vi "Store Value in TDMS.vi"(6 "Value":variant, 7 "Prefix":string, 8 "Error In":errorcluster, 9 "channel name":string, 10 "group name":string, 11 "tdms file":refnum<k34>) -> (0 "Error Out":errorcluster, 1 "channel name out":string, 2 "group name out":string, 3 "tdms file out":refnum<k34>)   [LabVIEW 2019]
uses:
  <vilib>/Utility/Data Type/Type Definitions/Data Type.ctl
  <vilib>/Utility/Data Type/NI_Data Type.lvlib
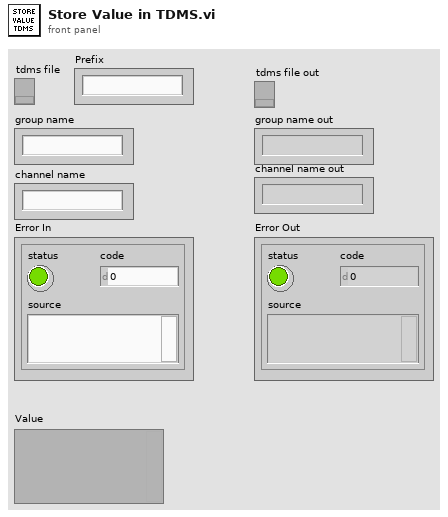
[diagram p1: front panel]
types:
  T1 = typedef "NI_Data Type.lvlib/Data Type.ctl" = enum8{"Invalid Type", "Void", "I8", "I16", "I32", "I64", "U8", "U16", "U32", "U64", "Single Float", "Double Float", "Extended Float", "Single Complex", "Double Complex", "Extended Complex", "Enum U8", "Enum U16", "Enum U32", "Enum U64", "Single Float With Unit", "Double Float With Unit", "Extended Float With Unit", "Single Complex with Unit", "Double Complex with Unit", "Extended Complex with Unit", "Boolean", "String", "Path", "Picture", "Tag", "Array", "Cluster", "Variant", "LV Variant", "Waveform", "Timestamp", "Digital Waveform", "Digital Data", "ExpressData", "Refnum", "External Data", "VI", "Poly VI", "LabVIEW Class Instance", "Fixed Point", "Set Collection", "Map Collection"}
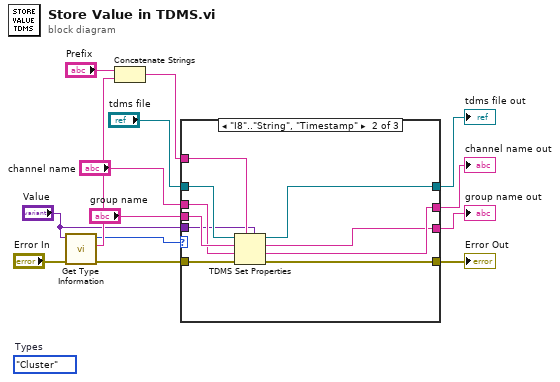
[diagram p0: block diagram]
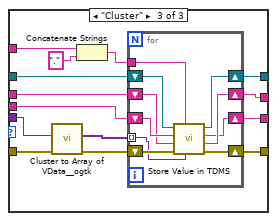
[diagram p3: hidden frame]
diagram:
  (unwired) Data_Type."Cluster"  # Types
  n1 = call <vilib>:"Get Type Information.vi"("error in (no error)"="Error In", "variant"="Value") -> ("error out"=w5:errorcluster, "name"=w7:string, "type"=w4:T1)  [unwired: 5 in, 2 out]
  n2 = Concatenate Strings("Prefix", w7) -> (w2:string)
  n3 = case shown="\"I8\"..\"String\", \"Timestamp\"" w4 {
    tunnel: "tdms file" -> [w18 w28 w42]
    tunnel: [w18 w27 w36] -> w13
    tunnel: "group name" -> [w16 w26 w41]
    tunnel: "channel name" -> [w15 w25 w40]
    tunnel: [w15 w24 w38] -> w10
    tunnel: [w16 w23 w39] -> w9
    tunnel: w5 -> [w17 w22 w30]
    tunnel: [w17 w21 w37] -> w8
    tunnel: w2 -> [_ w20 w35]
    tunnel: "Value" -> [_ w19 w32]
    frame "Invalid Type", Default {
    }
    frame "I8".."String", "Timestamp" {
      n4 = TDMS Set Properties(5:w19, 7:w20, 8:w22, 9:w25, 10:w26, 11:w28) -> (0:w21:errorcluster, 1:w24:string, 2:w23:string, 3:w27:refnum<k34>)
    }
    frame "Cluster" {
      n5 = call <userlib>:"Cluster to Array of VData__ogtk.vi"("error in (no error)"=w30, "Cluster"=w32) -> ("error out"=w29:errorcluster, "Array of VData"=w31:variant[])  [unwired: 8 in]
      n6 = Concatenate Strings(w35, "." ("string")) -> (w33:string)
      n7 = for {
        shift-right: [w49] -> w37
        shift-left: w29 -> [w51]
        shift-right: [w50] -> w36
        shift-left: w42 -> [w52]
        shift-right: [w45] -> w39
        shift-left: w41 -> [w48]
        shift-right: [w46] -> w38
        shift-left: w40 -> [w47]
        tunnel: w31 -> [w44] mode=indexing
        tunnel: w33 -> [w43]
        n8 = call "Store Value in TDMS.vi"("Value"=w44, "Prefix"=w43, "Error In"=w51, "channel name"=w47, "group name"=w48, "tdms file"=w52) -> ("Error Out"=w49:errorcluster, "channel name out"=w46:string, "group name out"=w45:string, "tdms file out"=w50:refnum<k34>)  [unwired: 2 in]
      }
    }
  }
  "Error Out" <- w8
  "tdms file out" <- w13
  "channel name out" <- w10
  "group name out" <- w9
